vi "I32 to HEX 8bits(SubVI).vi"(11 "IN U64":u64) -> (3 "OUT HEX 8BITS":string)   [LabVIEW 2014, in "CAP-USB.lvlib"]
doc: "Convierte la entrada U64 a un numero HEX\nde 8 bits"
uses:
  CAP-USB.lvlib
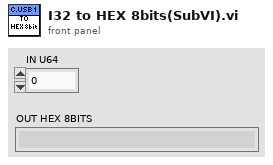
[diagram p1: front panel]
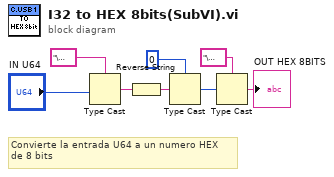
[diagram p0: block diagram]
diagram:
  # "Convierte la entrada U64 a un numero HEX\nde 8 bits"
  n1 = Type Cast(type="\u0000" ("string"), x="IN U64") -> (*(type *) &x=w6:string)
  n2 = Reverse String(1:w6) -> (0:w5:string)
  n3 = Type Cast(type=u8 0 ("y"), x=w5) -> (*(type *) &x=w3:u8)
  n4 = Type Cast(type="\u0000" ("string"), x=w3) -> (*(type *) &x=→"OUT HEX 8BITS":string)
